vi "Server Loop Async.vi"(11 "Websocket Server in":refnum<class "Websocket Server.lvclass">) -> ()   [LabVIEW 2020, in "Stream-Websocket.lvlib" / "Websocket Server.lvclass"]
uses:
  Websocket Server.lvclass
  C:/Program Files (x86)/National Instruments/LabVIEW 2020/vi.lib/IlluminatedG/lv-stream/Endpoint/Endpoint.lvclass
  Websocket Server.lvclass/Websocket Server.ctl
  <vilib>/IlluminatedG/lv-stream/Endpoint/Endpoint.lvclass
  Websocket Client/Websocket Client.lvclass
  C:/dev/IlluminatedG/lv-stream-websocket/Stream-Websocket/Websocket Server/Websocket Server.lvclass
panel:
  out "URI":string
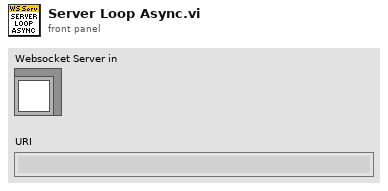
[diagram p1: front panel]
types:
  T1 = typedef "Stream-Websocket.lvlib/Listener Result.ctl" = cluster{"Status":T2, "Client":refnum<class "Websocket Client.lvclass">}
  T2 = typedef "Stream-Websocket.lvlib/Listener Status.ctl" = enum16{"Successful", "Unsuccessful"}
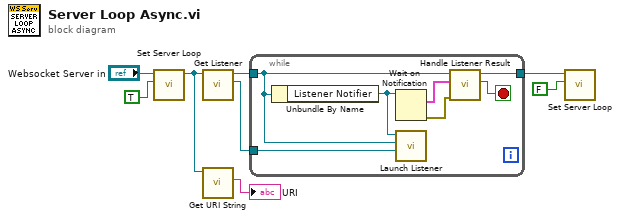
[diagram p0: block diagram]
diagram:
  n1 = call "Set Server Loop.vi"("Server Loop"=TRUE, "Websocket Server in"="Websocket Server in") -> ("Websocket Server out"=w6:refnum<class "Websocket Server.lvclass">)  [unwired: 8 in, 1 out]
  n2 = call "Get Listener.vi"("Websocket Server in"=w6) -> ("Listener"=w3:refnum<k5>, "Websocket Server out"=w4:refnum<class "Websocket Server.lvclass">)  [unwired: 8 in, 1 out]
  n3 = call <vilib>:"Get URI String.vi"("Endpoint in"=w6) -> ("URI String"=→"URI":string)  [unwired: 8 in, 2 out]
  n4 = while {
    tunnel: w4 -> [w9]
    tunnel: w3 -> [w10]
    tunnel: [w13] -> w2
    stop <- w12 stop-if-true
    n5 = Unbundle By Name(w9) -> ("Listener Notifier"=w11:refnum<notifier>)
    n6 = Wait on Notification(notifier=w11) -> (notification=w15:T1, error out=w14:errorcluster)  [unwired: 3 in, 2 out]
    n7 = call "Launch Listener.vi"("Listener"=w10, "Server Endpoint"=w9, "Listener Notifier"=w11) -> ()  [unwired: 8 in, 1 out]
    n8 = call "Handle Listener Result.vi"("error in (no error)"=w14, "Listener Result"=w15, "Websocket Server in"=w9) -> ("Shutdown"=w12:bool, "Websocket Server out"=w13:refnum<class "Websocket Server.lvclass">)  [unwired: 6 in, 1 out]
  }
  n9 = call "Set Server Loop.vi"("Server Loop"=FALSE, "Websocket Server in"=w2) -> ()  [unwired: 8 in, 2 out]
